vi "load waveforms.vi"(1 "waveform":path) -> (0 "# of points":i32)   [LabVIEW 2015]
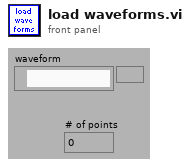
[diagram p1: front panel]
types:
  T1 = cluster{"AO parameters":cluster{"Build analog waveform tabs":dbl, "Repeats":dbl, "Cycles":dbl, "Start amplitude (V)":dbl, "Baseline (V)":dbl, "Step size (V)":dbl, "DC (%)":dbl, "Sampling frequency (Hz)":dbl, "Period (ms)":dbl, "Offset (V)":dbl, "Amplitude (V)":dbl, "Frequency":dbl, "Tri Repeats":dbl, "Cycle length (s)":dbl, "Pulses":dbl, "Matlab wave number":dbl}[], "DO parameters":cluster{"Digital DC (%)":dbl, "Digital phase":dbl, "Digital Freq (Hz)":dbl, "Sampling frequency (Hz)":dbl}[]}
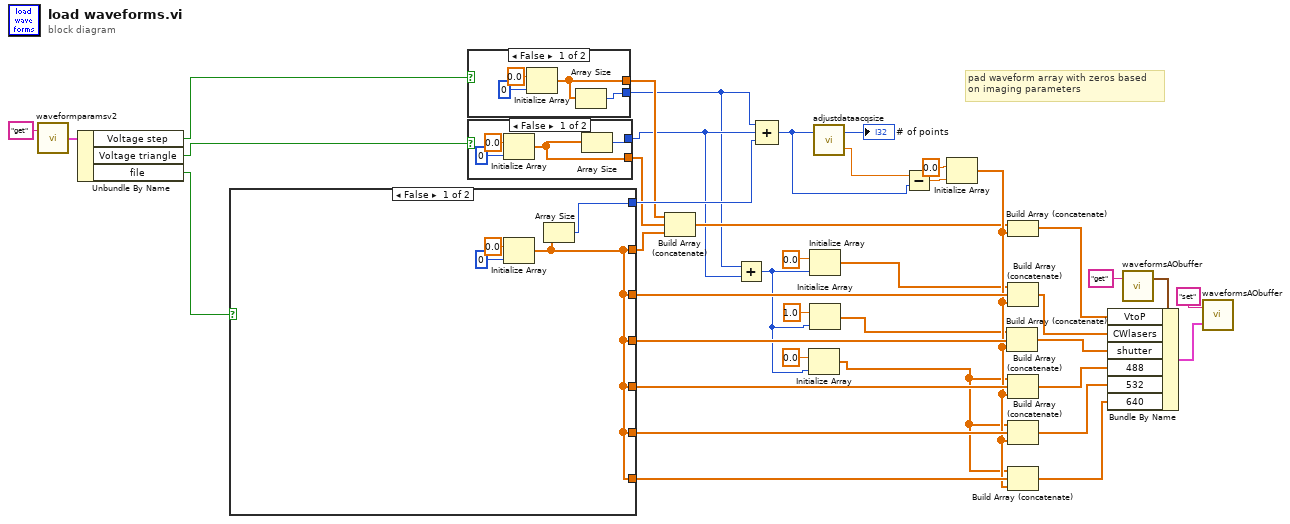
[diagram p0: block diagram]
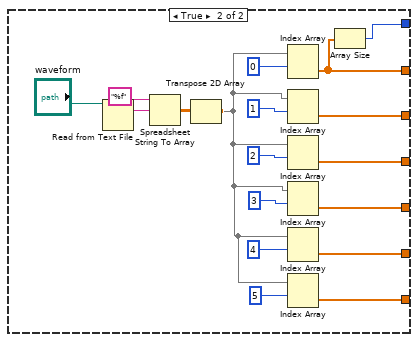
[diagram p2: hidden frame]
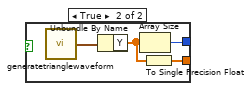
[diagram p3: hidden frame]
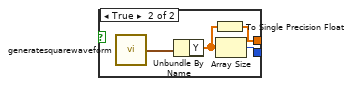
[diagram p4: hidden frame]
diagram:
  # "pad waveform array with zeros based\non imaging parameters"
  n1 = call "waveformparamsv2.vi"("command"="get") -> ("Params out"=w21:T1)  [unwired: 1 in]
  n2 = Unbundle By Name(w21) -> ("Voltage step"=w20:bool, "Voltage triangle"=w19:bool, "file"=w18:bool)
  n3 = case shown="False" w18 {
    tunnel: [w41 w62] -> w37
    tunnel: [w41 w61] -> w36
    tunnel: [w41 w60] -> w13
    tunnel: [w42 w53] -> w17
    tunnel: [w41 w47] -> w29
    tunnel: [w41 w46] -> w28
    tunnel: [w41 w45] -> w27
    frame False {
      n4 = Initialize Array(sgl 0.0 ("element"), 0 ("dimension size")) -> (w41:sgl[])
      n5 = Array Size(array=w41) -> (size(s)=w42:i32)
    }
    frame True {
      n6 = Read from Text File(file (use dialog)="waveform") -> (text=w59:string)  [unwired: 3 in, 3 out]
      n7 = Spreadsheet String To Array(format string="%f", spreadsheet string=w59) -> (array=w57:dbl[][])  [unwired: 2 in]
      n8 = Transpose 2D Array(2D array=w57) -> (transposed array=w48:dbl[][])
      n9 = Index Array(array=w48, index (row)=0) -> (element=w60:dbl[])  [unwired: 1 in]
      n10 = Index Array(array=w48, index (row)=1) -> (element=w61:dbl[])  [unwired: 1 in]
      n11 = Index Array(array=w48, index (row)=2) -> (element=w62:dbl[])  [unwired: 1 in]
      n12 = Index Array(array=w48, index (row)=3) -> (element=w46:dbl[])  [unwired: 1 in]
      n13 = Index Array(array=w48, index (row)=4) -> (element=w45:dbl[])  [unwired: 1 in]
      n14 = Index Array(array=w48, index (row)=5) -> (element=w47:dbl[])  [unwired: 1 in]
      n15 = Array Size(array=w60) -> (size(s)=w53:i32)
    }
  }
  n16 = case shown="False" w20 {
    tunnel: [w64 w67] -> w11
    tunnel: [w63 w68] -> w7
    frame False {
      n17 = Initialize Array(sgl 0.0 ("element"), 0 ("dimension size")) -> (w64:sgl[])
      n18 = Array Size(array=w64) -> (size(s)=w63:i32)
    }
    frame True {
      n19 = call "generatesquarewaveform.vi"() -> ("Waveform"=w70:waveform(dbl))  [unwired: 1 in]
      n20 = Unbundle By Name(w70) -> ("Y"=w69:dbl[])
      n21 = To Single Precision Float(number=w69) -> (single precision float=w67:sgl[])
      n22 = Array Size(array=w69) -> (size(s)=w68:i32)
    }
  }
  n23 = case shown="False" w19 {
    tunnel: [w71 w77] -> w8
    tunnel: [w72 w75] -> w12
    frame False {
      n24 = Initialize Array(sgl 0.0 ("element"), 0 ("dimension size")) -> (w72:sgl[])
      n25 = Array Size(array=w72) -> (size(s)=w71:i32)
    }
    frame True {
      n26 = call "generatetrianglewaveform.vi"() -> ("Waveform"=w78:waveform(dbl))  [unwired: 1 in]
      n27 = Unbundle By Name(w78) -> ("Y"=w76:dbl[])
      n28 = Array Size(array=w76) -> (size(s)=w77:i32)
      n29 = To Single Precision Float(number=w76) -> (single precision float=w75:sgl[])
    }
  }
  n30 = Build Array (concatenate)(w11, w12, w13) -> (w10:dbl[])
  n31 = Add(x=w7, y=w8) -> (x+y=w1:i32)
  n32 = Compound Arithmetic op=ADD(w7, w8, w17) -> (w16:i32)
  n33 = Initialize Array(sgl 0.0 ("element"), w1) -> (w2:sgl[])
  n34 = Initialize Array(sgl 0.0 ("element"), w1) -> (w6:sgl[])
  n35 = Initialize Array(sgl 1.0 ("element"), w1) -> (w4:sgl[])
  n36 = call "adjustdataacqsize.vi"("waveform size in"=w16) -> ("waveform size out"=w14:dbl, "# of points"=→"# of points":i32)  [unwired: 1 in]
  n37 = Subtract(x=w14, y=w16) -> (x-y=w34:dbl)
  n38 = Initialize Array(sgl 0.0 ("element"), w34) -> (w26:sgl[])
  n39 = Build Array (concatenate)(w4, w37, w26) -> (w40:dbl[])
  n40 = Build Array (concatenate)(w10, w26) -> (w38:dbl[])
  n41 = Build Array (concatenate)(w6, w36, w26) -> (w39:dbl[])
  n42 = Build Array (concatenate)(w2, w28, w26) -> (w25:dbl[])
  n43 = Build Array (concatenate)(w2, w27, w26) -> (w24:dbl[])
  n44 = Build Array (concatenate)(w2, w29, w26) -> (w23:dbl[])
  n45 = call "waveformsAObuffer.vi"("command"="get") -> ("AO wf out"=w31:waveform(dbl)[])  [unwired: 1 in]
  n46 = Bundle By Name(cluster=w31, "VtoP"=w38, "CWlasers"=w39, "shutter"=w40, "488"=w25, "532"=w24, "640"=w23) -> (w33:cluster{})
  n47 = call "waveformsAObuffer.vi"("AO wf in"=w33, "command"="set") -> ()  [unwired: 1 out]
